vi "SourceMeter.vi"(8 "error in (no error)":errorcluster) -> (0 "error out":errorcluster)   [LabVIEW 2018]
uses:
  classes/Tushars Events Toolkit/Software/Modules/EventClient_ObjectReference.ctl
  classes/Variable Manager/VariableManager_Bool.vi
  classes/Variable Manager/VariableManager_Double.vi
  ThirdParty/Keithley 24XX/Keithley 24XX.lvlib
  Strict Type Controls/Settings Operation.ctl
panel:
  out "scanTime(ms)":u32
  out "VIR":dbl[](array[numeric])
  out "Quit":bool
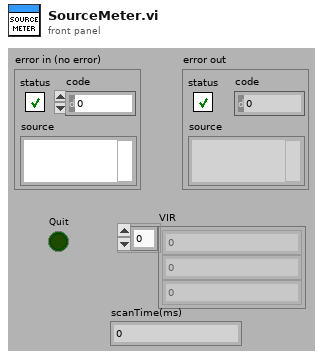
[diagram p1: front panel]
types:
  T1 = typedef "Settings Operation.ctl" = enum8{"Get Value", "Set Value", "Read File", "Write File", "Write Stored Value"}
  T2 = cluster{"Keithley":refnum<visa-resource-name>, "lastUpdate":u32}
  T3 = typedef "EventClient_ObjectReference.ctl" = refnum<k1>
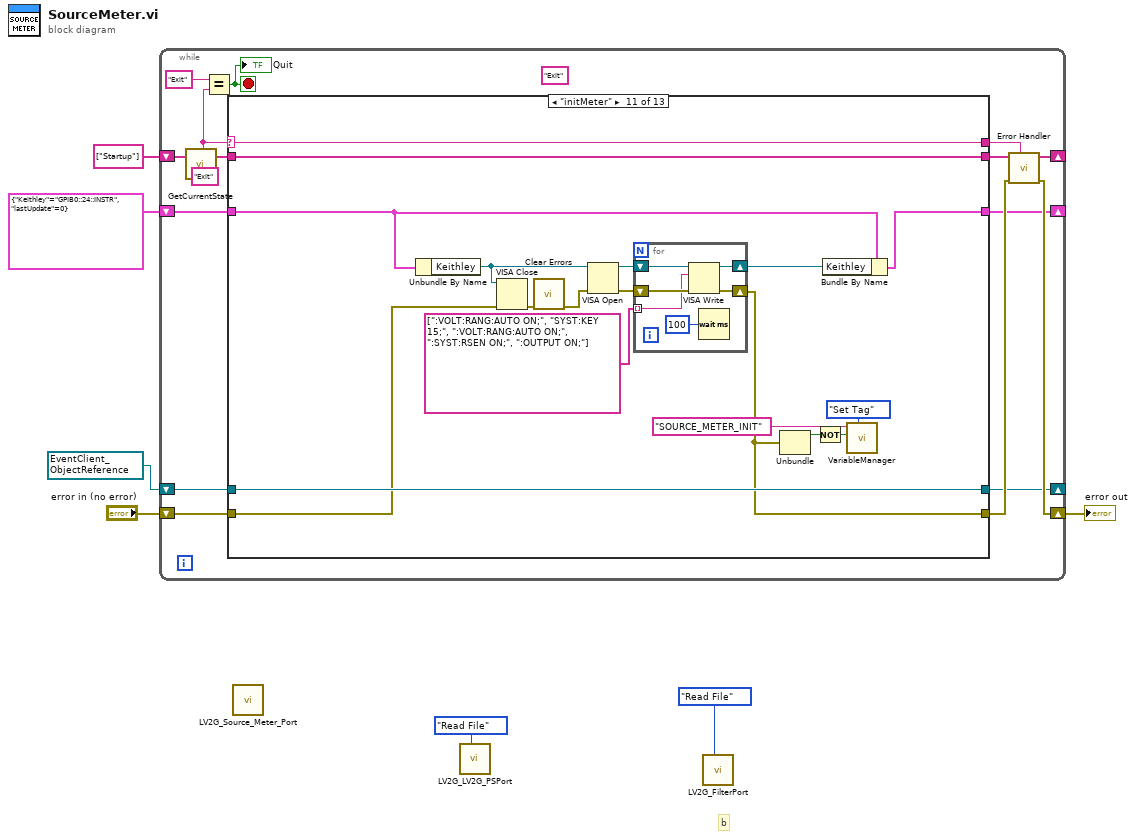
[diagram p0: block diagram]
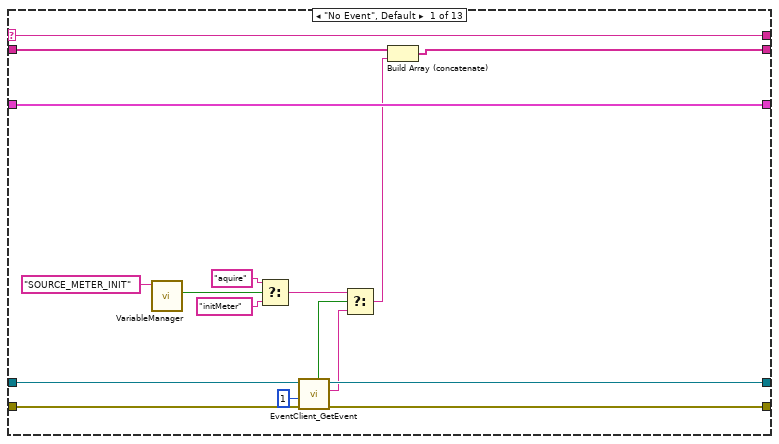
[diagram p2: hidden frame]
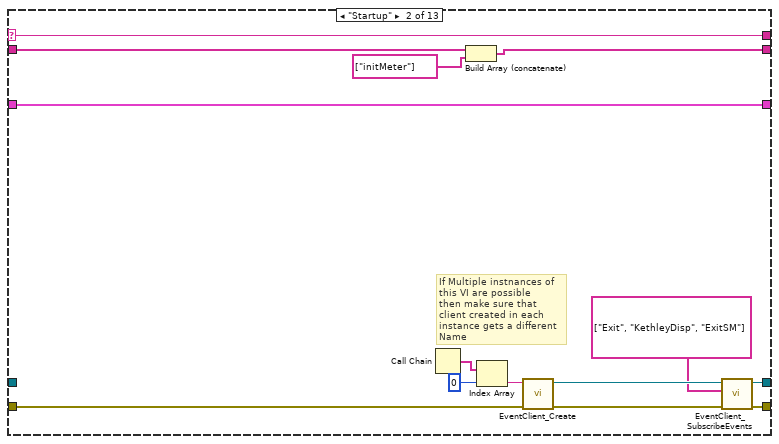
[diagram p3: hidden frame]
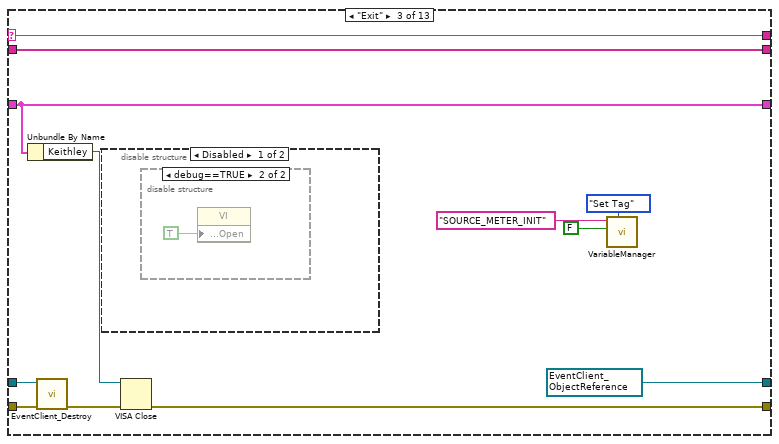
[diagram p4: hidden frame]
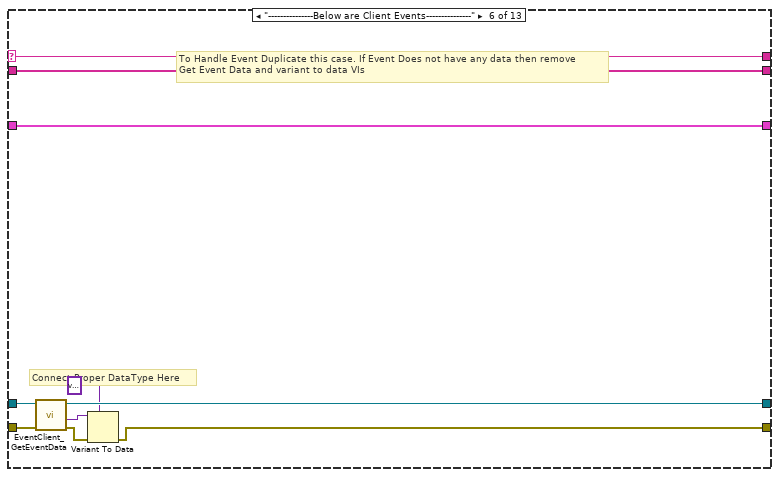
[diagram p9: hidden frame]
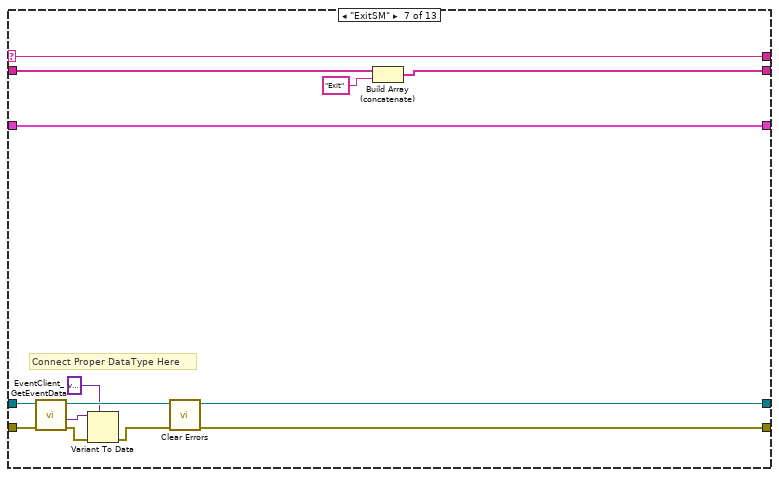
[diagram p10: hidden frame]
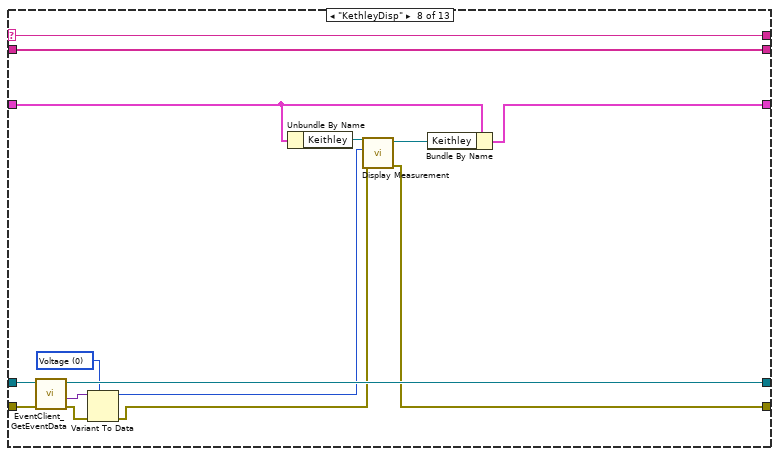
[diagram p11: hidden frame]
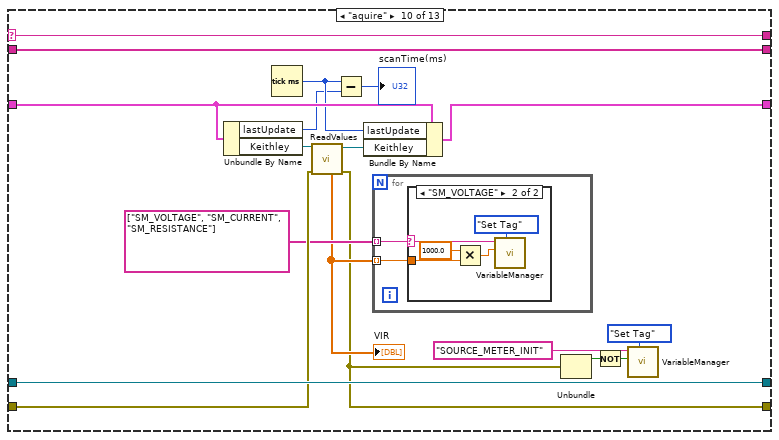
[diagram p13: hidden frame]
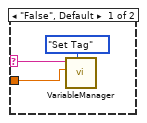
[diagram p14: hidden frame]
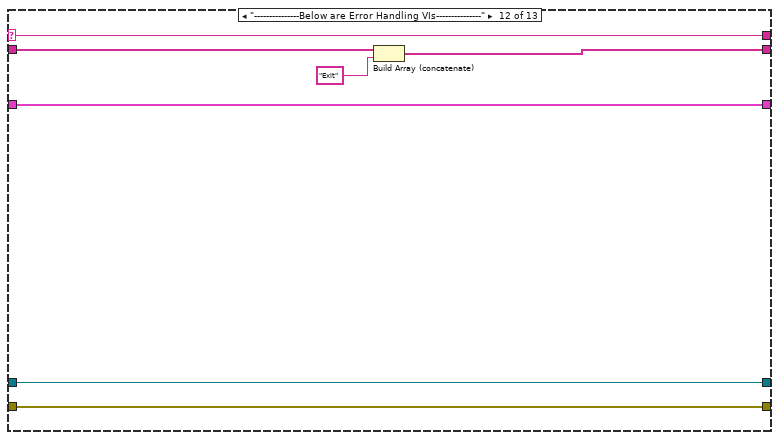
[diagram p15: hidden frame]
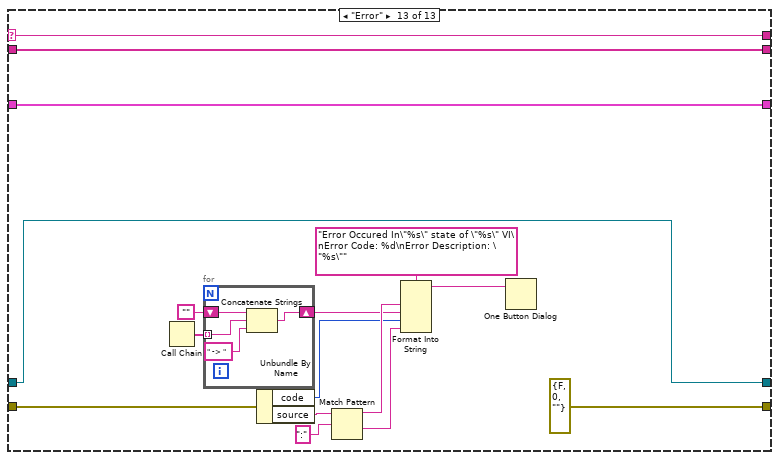
[diagram p16: hidden frame]
diagram:
  w4 = T3 refnum items=["EventClient"] ("reference")
  # "b"
  n1 = while {
    shift-right: [w18] -> _
    shift-left: string[] ["Startup"] ("State Array Out") -> [w22]
    shift-right: [w14] -> w5
    shift-left: "error in (no error)" -> [w15]
    shift-right: [w11] -> _
    shift-left: w4 -> [w10]
    shift-right: [w8] -> _
    shift-left: T2 {"Keithley"="GPIB0::24::INSTR", "lastUpdate"=0} -> [w9]
    stop <- w19 stop-if-true
    (unwired) "Exit" ("x")
    (unwired) "Exit" ("x")
    n2 = call "GetCurrentState.vi"("State Array In"=w22) -> ("Current State"=w12:string, "State Array Out"=w21:string[])  [unwired: 17 in]
    n3 = Equal?(x="Exit", y=w12) -> (x = y?=w19:bool)
    "Quit" <- w19
    n4 = case shown="\"initMeter\"" w12 {
      selector: w12 -> [w39 w53 w65 w70 w75 w85 w98 w113 w118 w136 w164 w178 w194]
      tunnel: w21 -> [w30 w52 w64 w71 w76 w86 w99 w114 w119 w137 w165 w177 w181]
      tunnel: [w34 w51 w64 w71 w76 w86 w89 w114 w119 w137 w165 w173 w181] -> w17
      tunnel: [w36 w44 w59 w69 w74 w81 w87 w101 w117 w124 w151 w176 errorcluster {"status"=FALSE, "code"=0, "source"=""} ("error in (no error)")] -> w13
      tunnel: [w39 w53 w65 w70 w75 w85 w98 w113 w118 w136 w164 w178 w194] -> w16
      tunnel: w15 -> [w37 w49 w62 w69 w74 w83 w96 w111 w117 w130 w154 w176 w182]
      tunnel: [w35 w42 w61 w68 w73 w79 w92 w108 w116 w135 w163 w175 w180] -> w11
      tunnel: w10 -> [w38 _ w63 w68 w73 w84 w97 w112 w116 w135 w163 w175 w180]
      tunnel: w9 -> [w32 w40 w58 w67 w72 w77 w90 w100 w115 w131 w159 w174 w179]
      tunnel: [w32 w40 w58 w67 w72 w77 w90 w105 w115 w132 w158 w174 w179] -> w8
      frame "No Event", Default {
        n5 = call-poly "VariableManager.vi"("Tag"="SOURCE_METER_INIT") -> ("Value out"=w26:bool)  [unwired: 7 in, 3 out]
        n6 = Select(t="aquire" ("Tag"), s=w26, f="initMeter" ("Tag")) -> (s? t:f=w23:string)
        n7 = call "EventClient_GetEvent.vi"("error in (no error)"=w37, "timeout in ms (-1)"=1, "reference"=w38) -> ("error out"=w36:errorcluster, "Name"=w28:string, "reference out"=w35:T3, "timed out?"=w29:bool)  [unwired: 4 in, 1 out]
        n8 = Select(t=w23, s=w29, f=w28) -> (s? t:f=w27:string)
        n9 = Build Array (concatenate)(w30, w27) -> (w34:string[])
      }
      frame "Startup" {
        # "If Multiple instnances of this VI are possible \nthen make sure that client created in each instance gets a different Name"
        n10 = Call Chain() -> (call chain=w48:string[])
        n11 = Build Array (concatenate)(w52, string[] ["initMeter"] ("State Array Out")) -> (w51:string[])
        n12 = Index Array(array=w48, index=0) -> (element=w46:string)
        n13 = call "EventClient_Create.vi"("error in (no error)"=w49, "Instance Name"=w46) -> ("error out"=w45:errorcluster, "reference"=w43:T3)  [unwired: 8 in]
        n14 = call "EventClient_SubscribeEvents.vi"("error in (no error)"=w45, "Events"=string[] ["Exit", "KethleyDisp", "ExitSM"], "reference"=w43) -> ("error out"=w44:errorcluster, "reference out"=w42:T3)  [unwired: 7 in]
      }
      frame "Exit" {
        w61 = T3 refnum items=["EventClient"] ("reference out")
        n15 = Unbundle By Name(w58) -> ("Keithley"=w57:refnum<visa-resource-name>)
        n16 = call "EventClient_Destroy.vi"("error in (no error)"=w62, "reference"=w63) -> ("error out"=w60:errorcluster)  [unwired: 9 in]
        n17 = disable-structure shown="Disabled" {
          frame Disabled {
            n18 = disable-structure shown="debug==TRUE" {
              frame condition #0 (active) {
              }
              frame condition #1 {
                n19 = property class="VI"("Front Panel.Open"=TRUE ("Front Panel Window:Open")) -> ()  [unwired: 2 in, 2 out]
              }
            }
          }
          frame Enabled {
          }
        }
        n20 = VISA Close(VISA resource name=w57, error in (no error)=w60) -> (error out=w59:errorcluster)
        n21 = call-poly "VariableManager.vi"("Operation"=enum16{"Get Tag", "Set Tag"}."Set Tag", "Value"=FALSE, "Tag"="SOURCE_METER_INIT") -> ()  [unwired: 5 in, 4 out]
      }
      frame "---------------Below are UI Events---------------" {
        # "This State will never Execute\nIt is added just for improving code readability please do not remove this case"
      }
      frame "---------------Below are Menu Events---------------" {
        # "This State will never Execute\nIt is added just for improving code readability please do not remove this case"
      }
      frame "---------------Below are Client Events---------------" {
        # "To Handle Event Duplicate this case. If Event Does not have any data then remove\nGet Event Data and variant to data VIs"
        # "Connect Proper DataType Here"
        n22 = call "EventClient_GetEventData.vi"("error in (no error)"=w83, "reference"=w84) -> ("error out"=w82:errorcluster, "Data"=w80:variant, "reference out"=w79:T3)  [unwired: 7 in]
        n23 = Variant To Data(error in=w82, type=variant, Variant=w80) -> (error out=w81:errorcluster)  [unwired: 1 out]
      }
      frame "ExitSM" {
        # "Connect Proper DataType Here"
        n24 = call "EventClient_GetEventData.vi"("error in (no error)"=w96, "reference"=w97) -> ("error out"=w95:errorcluster, "Data"=w93:variant, "reference out"=w92:T3)  [unwired: 7 in]
        n25 = Variant To Data(error in=w95, type=variant, Variant=w93) -> (error out=w94:errorcluster)  [unwired: 1 out]
        n26 = call <vilib>:"Clear Errors.vi"("error in (no error)"=w94) -> ("error out"=w87:errorcluster)  [unwired: 5 in, 1 out]
        n27 = Build Array (concatenate)(w99, "Exit" ("x")) -> (w89:string[])
      }
      frame "KethleyDisp" {
        w107 = u16 0 items=["Voltage", "Current", "Resistance"] ("Displayed Measurement (0: Voltage)")
        n28 = call "EventClient_GetEventData.vi"("error in (no error)"=w111, "reference"=w112) -> ("error out"=w110:errorcluster, "Data"=w109:variant, "reference out"=w108:T3)  [unwired: 7 in]
        n29 = Variant To Data(error in=w110, type=w107, Variant=w109) -> (data=w103:u16, error out=w102:errorcluster)
        n30 = Unbundle By Name(w100) -> ("Keithley"=w106:refnum<visa-resource-name>)
        n31 = call "Display Measurement.vi"("error in (no error)"=w102, "Displayed Measurement (0: Voltage)"=w103, "VISA resource name"=w106) -> ("error out"=w101:errorcluster, "VISA resource name out"=w104:refnum<visa-resource-name>)  [unwired: 7 in]
        n32 = Bundle By Name(cluster=w100, "Keithley"=w104) -> (w105:T2)
      }
      frame "---------------Below are Subroutine states---------------" {
      }
      frame "aquire" {
        n33 = Unbundle By Name(w131) -> ("lastUpdate"=w121:u32, "Keithley"=w134:refnum<visa-resource-name>)
        n34 = Tick Count (ms)() -> (millisecond timer value=w122:u32)
        n35 = call "ReadValues.vi"("error in (no error)"=w130, "Port"=w134) -> ("error out"=w124:errorcluster, "port out"=w133:refnum<visa-resource-name>, "VIR"=w128:dbl[])  [unwired: 5 in, 2 out]
        "VIR" <- w128
        n36 = Subtract(x=w122, y=w121) -> (x-y=→"scanTime(ms)":u32)
        n37 = Bundle By Name(cluster=w131, "lastUpdate"=w122, "Keithley"=w133) -> (w132:T2)
        n38 = for {
          tunnel: string[] ["SM_VOLTAGE", "SM_CURRENT", "SM_RESISTANCE"] ("State Array Out") -> [w138] mode=indexing
          tunnel: w128 -> [w139] mode=indexing
          n39 = case shown="\"SM_VOLTAGE\"" w138 {
            selector: w138 -> [w140 w145]
            tunnel: w139 -> [w141 w146]
            frame "False", Default {
              n40 = call-poly "VariableManager.vi"("Operation"=enum16{"Get Tag", "Set Tag"}."Set Tag", "Value"=w141, "Tag"=w140) -> ()  [unwired: 4 in, 5 out]
            }
            frame "SM_VOLTAGE" {
              n41 = Multiply(x=1000.0, y=w146) -> (x*y=w144:dbl)
              n42 = call-poly "VariableManager.vi"("Operation"=enum16{"Get Tag", "Set Tag"}."Set Tag", "Value"=w144, "Tag"=w145) -> ()  [unwired: 4 in, 5 out]
            }
          }
        }
        n43 = Unbundle(w124) -> ("status"=w126:bool)  [unwired: 2 out]
        n44 = Not(x=w126) -> (.not. x?=w123:bool)
        n45 = call-poly "VariableManager.vi"("Operation"=enum16{"Get Tag", "Set Tag"}."Set Tag", "Value"=w123, "Tag"="SOURCE_METER_INIT") -> ()  [unwired: 5 in, 4 out]
      }
      frame "initMeter" {
        n46 = Unbundle By Name(w159) -> ("Keithley"=w153:refnum<visa-resource-name>)
        n47 = VISA Close(VISA resource name=w153, error in (no error)=w154) -> (error out=w156:errorcluster)
        n48 = call <vilib>:"Clear Errors.vi"("error in (no error)"=w156) -> ("error out"=w155:errorcluster)  [unwired: 5 in, 1 out]
        n49 = VISA Open(error in (no error)=w155, VISA resource name=w153) -> (VISA resource name=w161:refnum<visa-resource-name>, error out=w157:errorcluster)  [unwired: 3 in]
        n50 = for {
          shift-right: [w169] -> w151
          shift-left: w157 -> [w171]
          tunnel: string[] [":VOLT:RANG:AUTO ON;", "SYST:KEY 15;", ":VOLT:RANG:AUTO ON;", ":SYST:RSEN ON;", ":OUTPUT ON;"] -> [w168] mode=indexing
          shift-right: [w167] -> w160
          shift-left: w161 -> [w166]
          n51 = VISA Write(VISA resource name=w166, write buffer=w168, error in (no error)=w171) -> (VISA resource name out=w167:refnum<visa-resource-name>, error out=w169:errorcluster)  [unwired: 1 out]
          n52 = Wait (ms)(milliseconds to wait=u32 100) -> ()  [unwired: 1 out]
        }
        n53 = Unbundle(w151) -> ("status"=w150:bool)  [unwired: 2 out]
        n54 = Not(x=w150) -> (.not. x?=w148:bool)
        n55 = Bundle By Name(cluster=w159, "Keithley"=w160) -> (w158:T2)
        n56 = call-poly "VariableManager.vi"("Operation"=enum16{"Get Tag", "Set Tag"}."Set Tag", "Value"=w148, "Tag"="SOURCE_METER_INIT") -> ()  [unwired: 5 in, 4 out]
      }
      frame "---------------Below are Error Handling VIs---------------" {
        n57 = Build Array (concatenate)(w177, "Exit" ("x")) -> (w173:string[])
      }
      frame "Error" {
        n58 = Call Chain() -> (call chain=w189:string[])
        n59 = for {
          tunnel: w189 -> [w197] mode=indexing
          shift-right: [w195] -> w186
          shift-left: "" -> [w198]
          n60 = Concatenate Strings(w198, w197, " -> ") -> (w195:string)
        }
        n61 = Unbundle By Name(w182) -> ("code"=w184:i32, "source"=w183:string)
        n62 = Match Pattern(string=w183, regular expression=":") -> (before substring=w187:string, after substring=w191:string)  [unwired: 1 in, 2 out]
        n63 = Format Into String(format string="Error Occured In\"%s\" state of \"%s\" VI\nError Code: %d\nError Description: \"%s\"", w187, w186, w184, w191) -> (resulting string=w190:string)  [unwired: 2 in, 1 out]
        n64 = One Button Dialog(message=w190) -> ()  [unwired: 1 in, 1 out]
      }
    }
    n65 = call "Error Handler.vi"("Current State"=w16, "error in (no error)"=w13, "Msg Queue In"=w17) -> ("error out"=w14:errorcluster, "Msg Queue Out"=w18:string[])  [unwired: 7 in]
  }
  "error out" <- w5
  n66 = call "LV2G_Source_Meter_Port.vi"() -> ()  [unwired: 10 in, 2 out]
  n67 = call "LV2G_LV2G_PSPort.vi"("Operation"=Settings_Operation."Read File") -> ()  [unwired: 9 in, 2 out]
  n68 = call "LV2G_FilterPort.vi"("Operation"=Settings_Operation."Read File") -> ()  [unwired: 9 in, 2 out]
